vi "% span to Voltage 2 v1_0.vi"(2 "% span":dbl format="%.2f") -> (0 "Output Voltage":dbl format="%.2f")   [LabVIEW 2012]
panel:
  in  "Minimum Voltage":dbl format="%.2f"
  in  "Maximum Voltage":dbl=10.0 format="%.2f"
  # "% span to Voltage 2"
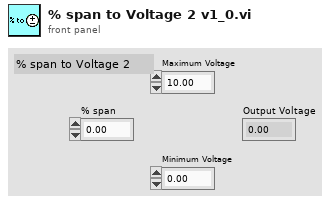
[diagram p1: front panel]
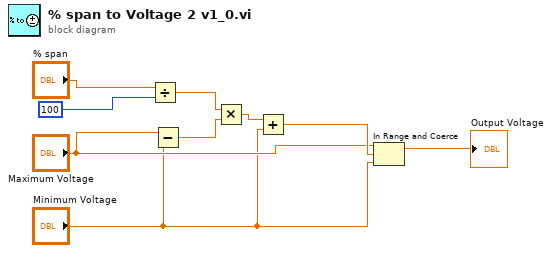
[diagram p0: block diagram]
diagram:
  n1 = Divide(x="% span", y=100) -> (x/y=w7:dbl)
  n2 = Subtract(x="Maximum Voltage", y="Minimum Voltage") -> (x-y=w6:dbl)
  n3 = Multiply(x=w7, y=w6) -> (x*y=w5:dbl)
  n4 = Add(x=w5, y="Minimum Voltage") -> (x+y=w4:dbl)
  n5 = In Range and Coerce(upper limit="Maximum Voltage", x=w4, lower limit="Minimum Voltage") -> (coerced(x)=→"Output Voltage":dbl)  [unwired: 1 out]
